vi "读取-数据库连接引用.vi"(8 "error in (no error)":errorcluster caption="错误输入（无错误）", 11 "数据库操作输入":refnum<class "数据库操作.lvclass">) -> (0 "error out":errorcluster caption="错误输出", 2 "reference":T1, 3 "数据库操作输出":refnum<class "数据库操作.lvclass">)   [LabVIEW 2013, in "数据库操作.lvclass"]
uses:
  <vilib>/addons/database/Connection.llb/Conn ObjectReference.ctl
  <vilib>/addons/database/NI_Database_API.lvlib
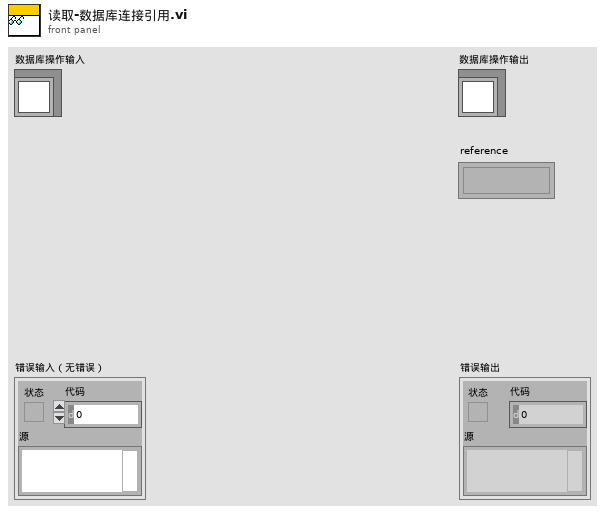
[diagram p1: front panel]
types:
  T1 = typedef "NI_Database_API.lvlib/Conn ObjectReference.ctl" = refnum<k1>
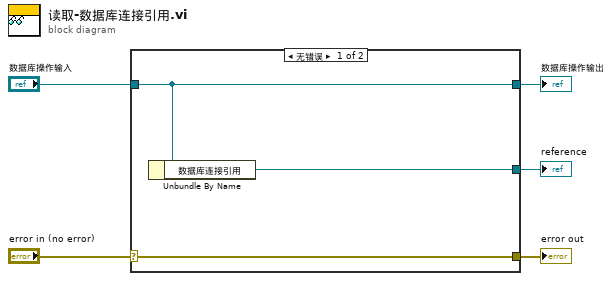
[diagram p0: block diagram]
diagram:
  n1 = case shown="无错误" "error in (no error)" {
    selector: "error in (no error)" -> [w8 w9]
    tunnel: [w8 w9] -> w4
    tunnel: [w7 w10] -> w2
    tunnel: "数据库操作输入" -> [w7 w10]
    tunnel: [w6 _] -> w1
    frame No Error {
      n2 = Unbundle By Name(w7) -> ("数据库连接引用"=w6:T1)
    }
    frame Error {
    }
  }
  "error out" <- w4
  "数据库操作输出" <- w2
  "reference" <- w1
